vi "pp_sessList_createPseudoGellerman.vi"(8 "error in (no error)":errorcluster, 10 "Total Trials":i32=15 min=3 step=1, 11 "Trial Types":T1(array[cluster])=[{"Trial Code"=1, "Trial Type"=enum."GO", "Trial Weight"=1, "Stim Type"=enum."FM Sweep", "Stim Dur (s)"=0.25, "Stim P1"=2000.0, "Stim P2"=4000.0}, {"Trial Code"=2, "Trial Type"=enum."NOGO", "Trial Weight"=1, "Stim Type"=enum."FM Sweep", "Stim Dur (s)"=0.25, "Stim P1"=4000.0, "Stim P2"=2000.0}, {"Trial Code"=3, "Trial Type"=enum."TEST", "Trial Weight"=1, "Stim Type"=enum."Pure Tone", "Stim Dur (s)"=0.25, "Stim P1"=400.0, "Stim P2"=0.0}] {"Stim P2" min=0.0; "Trial Weight" step=1; "Stim P1" min=0.0; "Stim Dur (s)" min=0.0; "Trial Code" min=1 step=1}) -> (0 "error out":errorcluster, 3 "Session List (Cannot Edit)":i32[](array[numeric]))   [LabVIEW 2013]
uses:
  labolabo/array/impl/NullArray_I.vi
  labolabo/random/impl/RandomizeArray_I.vi
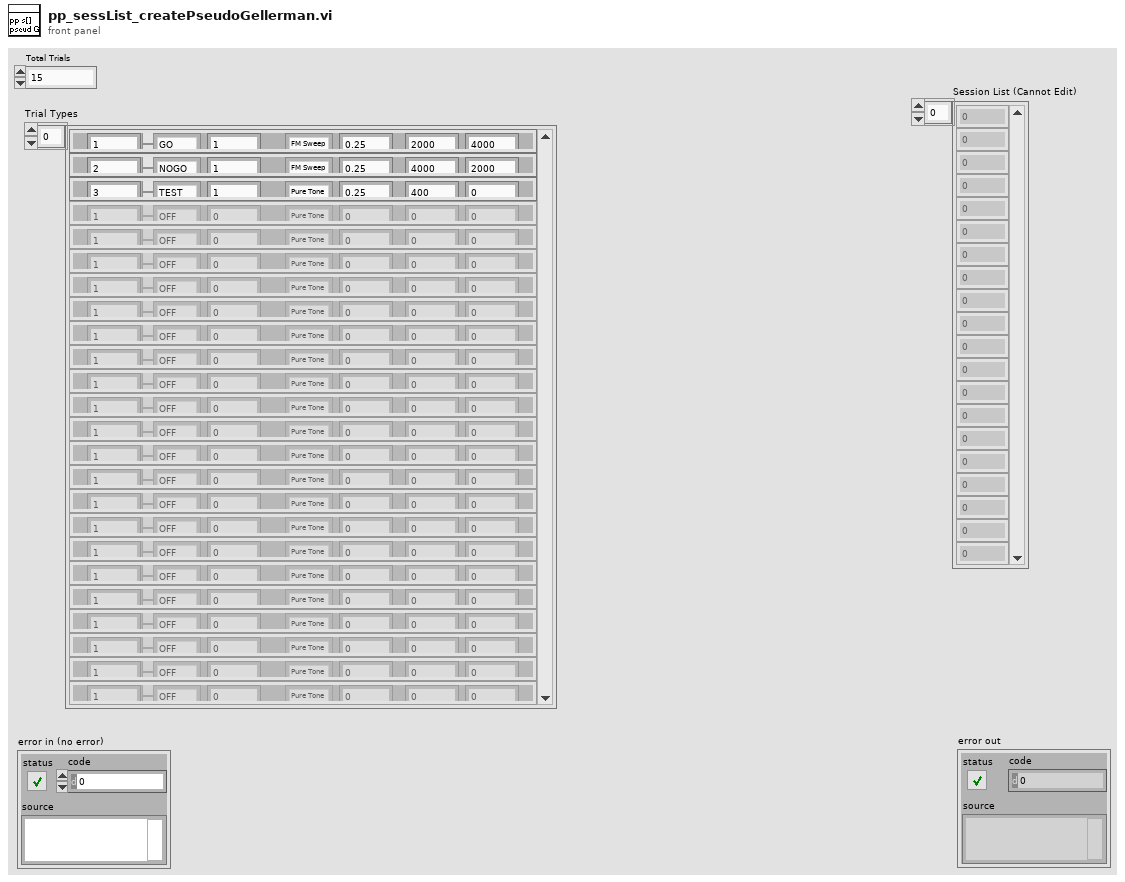
[diagram p1: front panel]
types:
  T1 = cluster{"Trial Code":u16, "Trial Type":enum16{"OFF", "GO", "NOGO", "TEST"}, "Trial Weight":u32, "Stim Type":enum16{"Pure Tone", "FM Sweep"}, "Stim Dur (s)":dbl, "Stim P1":dbl, "Stim P2":dbl}[]
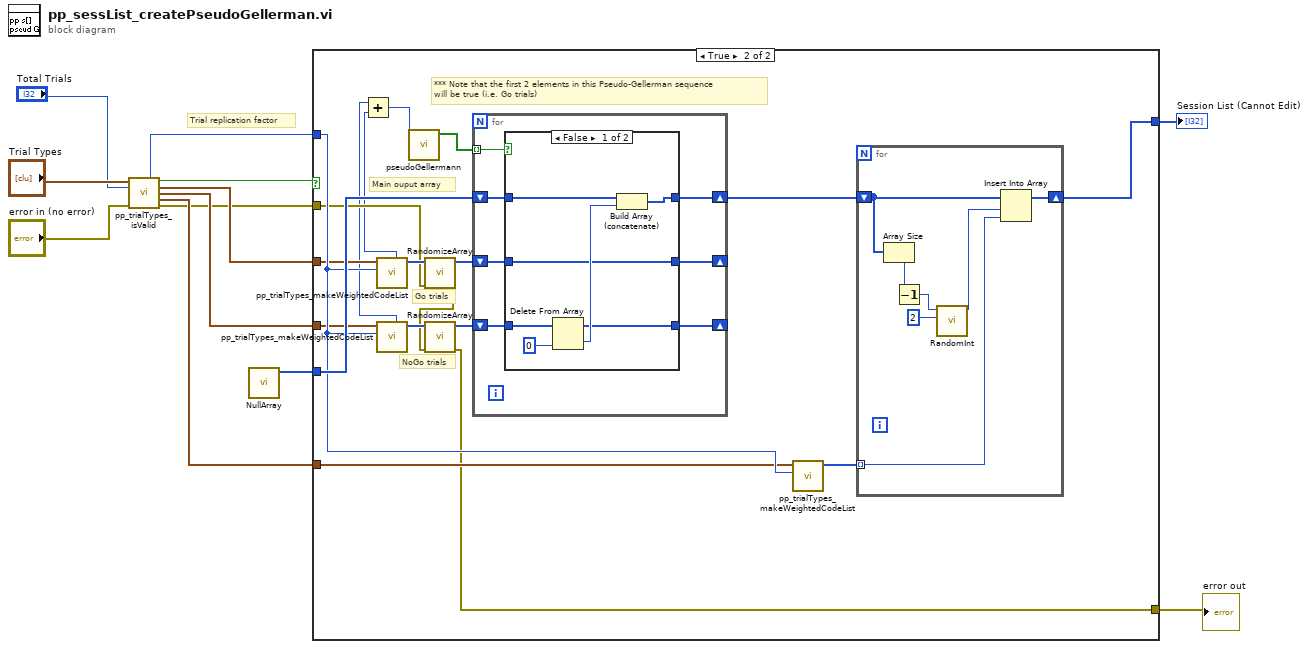
[diagram p0: block diagram]
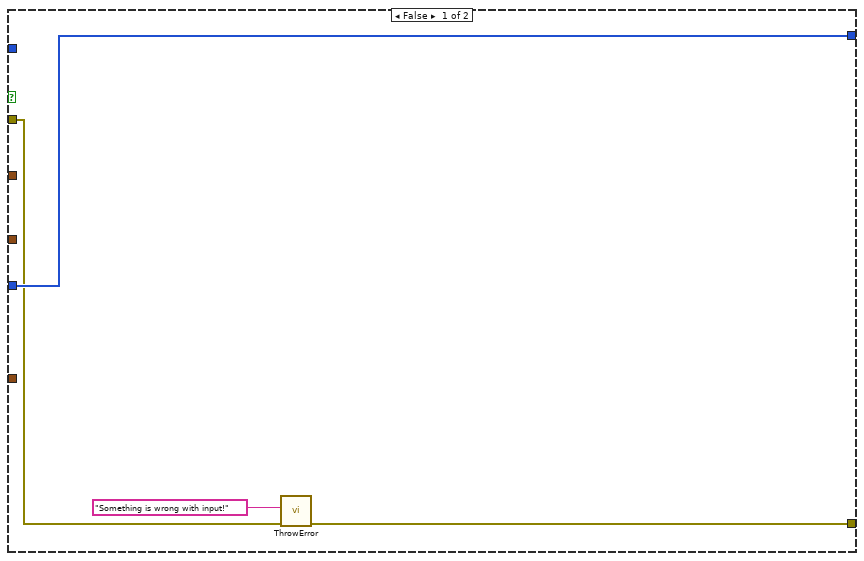
[diagram p2: hidden frame]
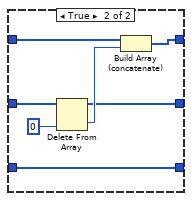
[diagram p3: hidden frame]
diagram:
  # "Trial replication factor"
  n1 = call "pp_trialTypes_isValid.vi"("Trial Types"="Trial Types", "Total Trials"="Total Trials", "error in (no error)"="error in (no error)") -> ("Trial Replication Factor"=w7:i32, "Paradigm Valid?"=w5:bool, "GO Trials"=w4:T1, "NOGO Trials"=w3:T1, "TEST Trials"=w2:T1, "error out"=w1:errorcluster)  [unwired: 7 in]
  n2 = call-poly "NullArray.vi"() -> ("Null Array"=w12:i32[])  [unwired: 11 in]
  n3 = case shown="True" w5 {
    tunnel: w7 -> [_ w27]
    tunnel: w12 -> [w16 w30]
    tunnel: [w16 w28] -> w11
    tunnel: [w14 w21] -> w10
    tunnel: w4 -> [_ w26]
    tunnel: w3 -> [_ w25]
    tunnel: w2 -> [_ w24]
    tunnel: w1 -> [w13 w23]
    frame False {
      n4 = call "ThrowError.vi"("error in (no error)"=w13, "Error Message"="Something is wrong with input!" ("error message (\"\")")) -> ("error out"=w14:errorcluster)  [unwired: 8 in, 1 out]
    }
    frame True {
      # "*** Note that the first 2 elements in this Pseudo-Gellerman sequence\nwill be true (i.e. Go trials)"
      # "NoGo trials"
      # "Go trials"
      # "Main ouput array"
      n5 = call "pp_trialTypes_makeWeightedCodeList.vi"("Trial Replication Factor"=w27, "Trial Types"=w26) -> ("Weighted Code List"=w33:i32[], "Weighted Code List Length"=w18:i32)  [unwired: 8 in]
      n6 = call "pp_trialTypes_makeWeightedCodeList.vi"("Trial Replication Factor"=w27, "Trial Types"=w25) -> ("Weighted Code List"=w32:i32[], "Weighted Code List Length"=w17:i32)  [unwired: 8 in]
      n7 = Add(x=w17, y=w18) -> (x+y=w19:i32)
      n8 = call "pseudoGellermann.vi"("N"=w19) -> ("Array"=w35:bool[])  [unwired: 10 in]
      n9 = call-poly "RandomizeArray.vi"("error in (no error)"=w23, "Array In"=w33) -> ("error out"=w22:errorcluster, "Array Out"=w34:i32[])  [unwired: 8 in]
      n10 = call-poly "RandomizeArray.vi"("error in (no error)"=w22, "Array In"=w32) -> ("error out"=w21:errorcluster, "Array Out"=w31:i32[])  [unwired: 8 in]
      n11 = for {
        tunnel: w35 -> [w49] mode=indexing
        shift-right: [w44] -> _
        shift-left: w34 -> [w45]
        shift-right: [w46] -> _
        shift-left: w31 -> [w47]
        shift-right: [w43] -> w29
        shift-left: w30 -> [w48]
        n12 = case shown="False" w49 {
          tunnel: [w55 w62] -> w43
          tunnel: w48 -> [w54 w61]
          tunnel: w47 -> [w52 w60]
          tunnel: [w51 w60] -> w46
          tunnel: w45 -> [w50 w59]
          tunnel: [w50 w57] -> w44
          frame False {
            n13 = Delete From Array(array=w52, index=0 ("index (row)")) -> (deleted portion=w53:i32, array with subset deleted=w51:i32[])  [unwired: 1 in]
            n14 = Build Array (concatenate)(w54, w53) -> (w55:i32[])
          }
          frame True {
            n15 = Delete From Array(array=w59, index=0 ("index (row)")) -> (deleted portion=w58:i32, array with subset deleted=w57:i32[])  [unwired: 1 in]
            n16 = Build Array (concatenate)(w61, w58) -> (w62:i32[])
          }
        }
      }
      n17 = call "pp_trialTypes_makeWeightedCodeList.vi"("Trial Replication Factor"=w27, "Trial Types"=w24) -> ("Weighted Code List"=w20:i32[])  [unwired: 8 in, 1 out]
      n18 = for {
        tunnel: w20 -> [w37] mode=indexing
        shift-right: [w38] -> w28
        shift-left: w29 -> [w39]
        n19 = Array Size(array=w39) -> (size(s)=w40:i32)
        n20 = Decrement(x=w40) -> (x-1=w41:i32)
        n21 = call "RandomInt.vi"("Min"=2, "Max"=w41) -> ("Random"=w36:i32)  [unwired: 9 in]
        n22 = Insert Into Array(array=w39, index=w36, new element=w37) -> (w38:i32[])
      }
    }
  }
  "error out" <- w10
  "Session List (Cannot Edit)" <- w11
